vi "fgv_AOL_Globals Write.vi"(8 "error in (no error)":errorcluster, 10 "AOL_Globals":T1={"Imaging Protocol"=enum."AOL Z-Stack", "Number of POI"=0, "Number of Miniscans"=0, "Number of Trials"=0, "Number of Cycles "=0, "# Averaged Frames"=0, "Laser power (%)"=0, "Pockels"=0.0, "Acquisition Length (sec)"=0.0, "Fill time (us)"=0.0, "POI Dwell time (us)"=0.0, "Miniscan Dwell time per pixel (us)"=0.0, "PMT 1"=0.0, "PMT 2"=0.0, "Back Apperture"=0.0, "Frame Size"=0, "Center Frequency"=0.0, "Field of View"=0.0, "DwellTime (us)"=0.0, "Wavelength (nm)"=0.0, "Zoom"=0.0, "AOL Z"=0.0, "AOL Mode"=enum."Raster", "GridXY"=0.0, "GridZ"=0.0, "TriggerPeriod (sec)"=0.0, "Number of Pixels in Miniscan"=0, "Experiment folder path"=path "", "X centre"=0.0, "Y centre"=0.0, "Angle (degrees)"=0.0, "Plane Mode"=0, "Threshold"=[], "Regenerate Chirps"=FALSE, "Rectangle ROI length (pixels)"=0, "Rectangle ROI height (pixels)"=0, "AOD fill"=0, "Samples Wait after Trigger"=0, "StartUp Delay"=0, "Slip Cycle"=163840, "Add Cycle"=FALSE} {"Plane Mode" items=["XY Plane"]; "Frame Size" items=["100X100"=100, "128X128"=128, "200X200"=200, "256X256"=256, "512X512"=512, "1024x1024"=1024, "2048x2048"=2048]; "Back Apperture" format="%#.6g"; "Pockels" format="%#.6g"; "PMT 2" format="%#.6g"; "PMT 1" format="%#.6g"; "Angle (degrees)" format="%#.6g"; "POI Dwell time (us)" format="%#.6g"}) -> (0 "error out":errorcluster)   [LabVIEW 2013]
uses:
  Typedefs/Controls/AOL_Globals.ctl
  Typedefs/Imaging Protocols enum.ctl
  Typedefs/Frame Size.ctl
  Typedefs/AOL modes.ctl
  Typedefs/Plane Mode.ctl
panel:
  out "delimited string":string
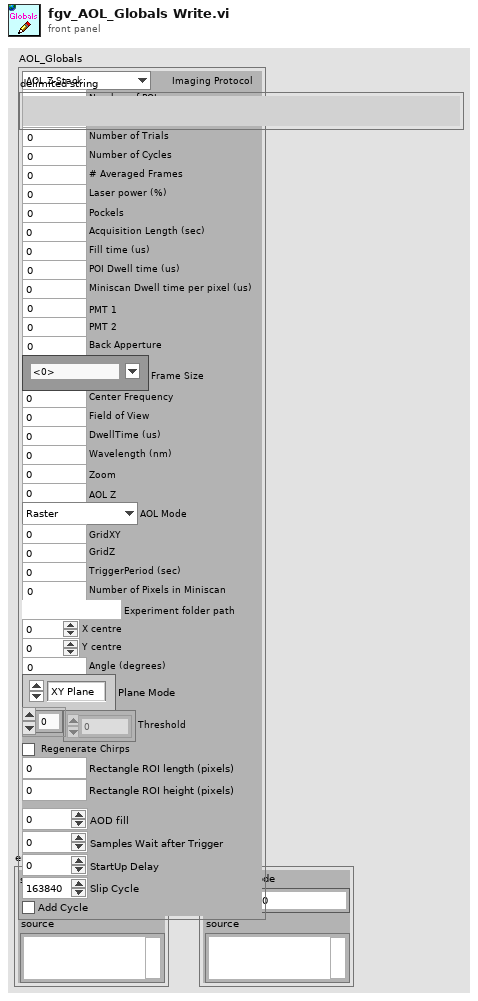
[diagram p1: front panel]
types:
  T1 = typedef "AOL_Globals.ctl" = cluster{"Imaging Protocol":T2, "Number of POI":u16, "Number of Miniscans":u16, "Number of Trials":u16, "Number of Cycles ":u64, "# Averaged Frames":u16, "Laser power (%)":u8, "Pockels":dbl, "Acquisition Length (sec)":dbl, "Fill time (us)":dbl, "POI Dwell time (us)":dbl, "Miniscan Dwell time per pixel (us)":dbl, "PMT 1":dbl, "PMT 2":dbl, "Back Apperture":dbl, "Frame Size":T3, "Center Frequency":dbl, "Field of View":dbl, "DwellTime (us)":dbl, "Wavelength (nm)":dbl, "Zoom":dbl, "AOL Z":dbl, "AOL Mode":T4, "GridXY":dbl, "GridZ":dbl, "TriggerPeriod (sec)":dbl, "Number of Pixels in Miniscan":u16, "Experiment folder path":path, "X centre":dbl, "Y centre":dbl, "Angle (degrees)":dbl, "Plane Mode":T5, "Threshold":u16[], "Regenerate Chirps":bool, "Rectangle ROI length (pixels)":u16, "Rectangle ROI height (pixels)":u16, "AOD fill":u16, "Samples Wait after Trigger":u16, "StartUp Delay":i32, "Slip Cycle":u32, "Add Cycle":bool}
  T2 = typedef "Imaging Protocols enum.ctl" = enum16{"AOL Z-Stack", "Motor Z Stack", "Functional Acquisition", "Single Plane Acquisition", "Volume Acquisition", "Live Imaging", "Live Plane Imaging", "Live Volume Imaging"}
  T3 = typedef "Frame Size.ctl" = u16
  T4 = typedef "AOL modes.ctl" = enum16{"Raster", "Structural", "Pointing", "Mini Scan", "Alignment"}
  T5 = typedef "Plane Mode.ctl" = u16
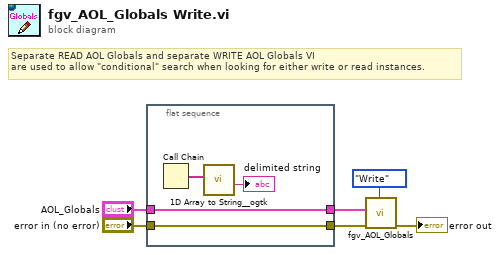
[diagram p0: block diagram]
diagram:
  # "Separate READ AOL Globals and separate WRITE AOL Globals VI \nare used to allow \"conditional\" search when looking for either write or read instances."
  n1 = flat-sequence {
    tunnel: [w8] -> w3
    tunnel: "error in (no error)" -> [w8]
    tunnel: [w7] -> w2
    tunnel: "AOL_Globals" -> [w7]
    frame #0 {
      n2 = Call Chain() -> (call chain=w10:string[])
      n3 = call <userlib>:"1D Array to String__ogtk.vi"("Array of Strings"=w10) -> ("delimited string"=→"delimited string":string)  [unwired: 10 in]
    }
  }
  n4 = call "fgv_AOL_Globals.vi"("error in (no error)"=w3, "AOL_Globals"=w2, "Function"=enum16{"Intialize", "Write", "Read", "Clear"}."Write") -> ("error out"=→"error out":errorcluster)  [unwired: 7 in, 1 out]
